vi "CD Init_Prepare Inline Data_Complete Frame Descriptors.vi"(8 "error in (no error)":errorcluster, 10 "RTs In":T1[](array[typedef]) {"Mode Codes"."Words Item Refs" format="%.0x"; "Mode Codes"."Words Block Data Refs"."Data Reference" format="%.0x"; "Mode Codes"."Timestamp Channel Data Reference" format="%.0x"; "subAddresses"."Words Item Refs" format="%.0x"; "subAddresses"."Words Block Data Refs"."Data Reference" format="%.0x"; "subAddresses"."Timestamp Channel Data Reference" format="%.0x"; "Status Channel Data Reference" format="%.0x"; "Command Channels Refs" format="%.0x"}, 11 "Frames Descriptors In":T9[](array[typedef]) {"RT"."Status Channel Ref" format="%.0x"; "RT"."Words Block Data Refs"."Data Reference" format="%.0x"; "RT"."Timestamp Channel Data Reference" format="%.0x"; "BC"."Status Channel Refs" format="%.0x"; "BC"."Words Block Data Refs"."Data Reference" format="%.0x"; "BC"."Timestamp Channel Data Reference" format="%.0x"}) -> (0 "error out":errorcluster, 3 "Frames Descriptors Out":T9[](array[typedef]) {"RT"."Status Channel Ref" format="%.0x"; "RT"."Words Block Data Refs"."Data Reference" format="%.0x"; "RT"."Timestamp Channel Data Reference" format="%.0x"; "BC"."Status Channel Refs" format="%.0x"; "BC"."Words Block Data Refs"."Data Reference" format="%.0x"; "BC"."Timestamp Channel Data Reference" format="%.0x"})   [LabVIEW 2017, in "Ballard MIL-1553 Engine.lvlib"]
doc: "We complete Frame Descriptors for frames not defined in BC (or there is no BC)."
uses:
  Ballard MIL-1553 Engine.lvlib
  Controls/RT Inline Frame Descriptor.ctl
  Controls/RT Inline Frame Descriptor_BC.ctl
  <vilib>/NI Veristand/Custom Device API/Data Reference.ctl
  <vilib>/NI Veristand/Custom Device API/Block Data Reference.ctl
  <vilib>/NI Veristand/Custom Device API/Custom Device Item Ref.ctl
  Controls/RT Inline Frame Descriptor_RT.ctl
  Shared/Controls and Global/RT CWD2.ctl
  Shared/Controls and Global/RT CWD1.ctl
  Shared/Controls and Global/RT messageType.ctl
  Shared/Controls and Global/RT Remote Terminal.ctl
  Shared/Controls and Global/RT Remote Terminal_rtMode.ctl
  Shared/Controls and Global/RT Remote Terminal_RT subAddress.ctl
  Shared/Controls and Global/RT Remote Terminal_RT direction.ctl
  Shared/Controls and Global/RT Remote Terminal_RT Mode Code.ctl
  <vilib>/NI VeriStand/Custom Device Tools/Custom Device Utility Library/Custom Device Utility Library.lvlib
  Shared/Ballard 1553 Shared.lvlib
  <vilib>/NI VeriStand/Custom Device API/Custom Device API.lvlib
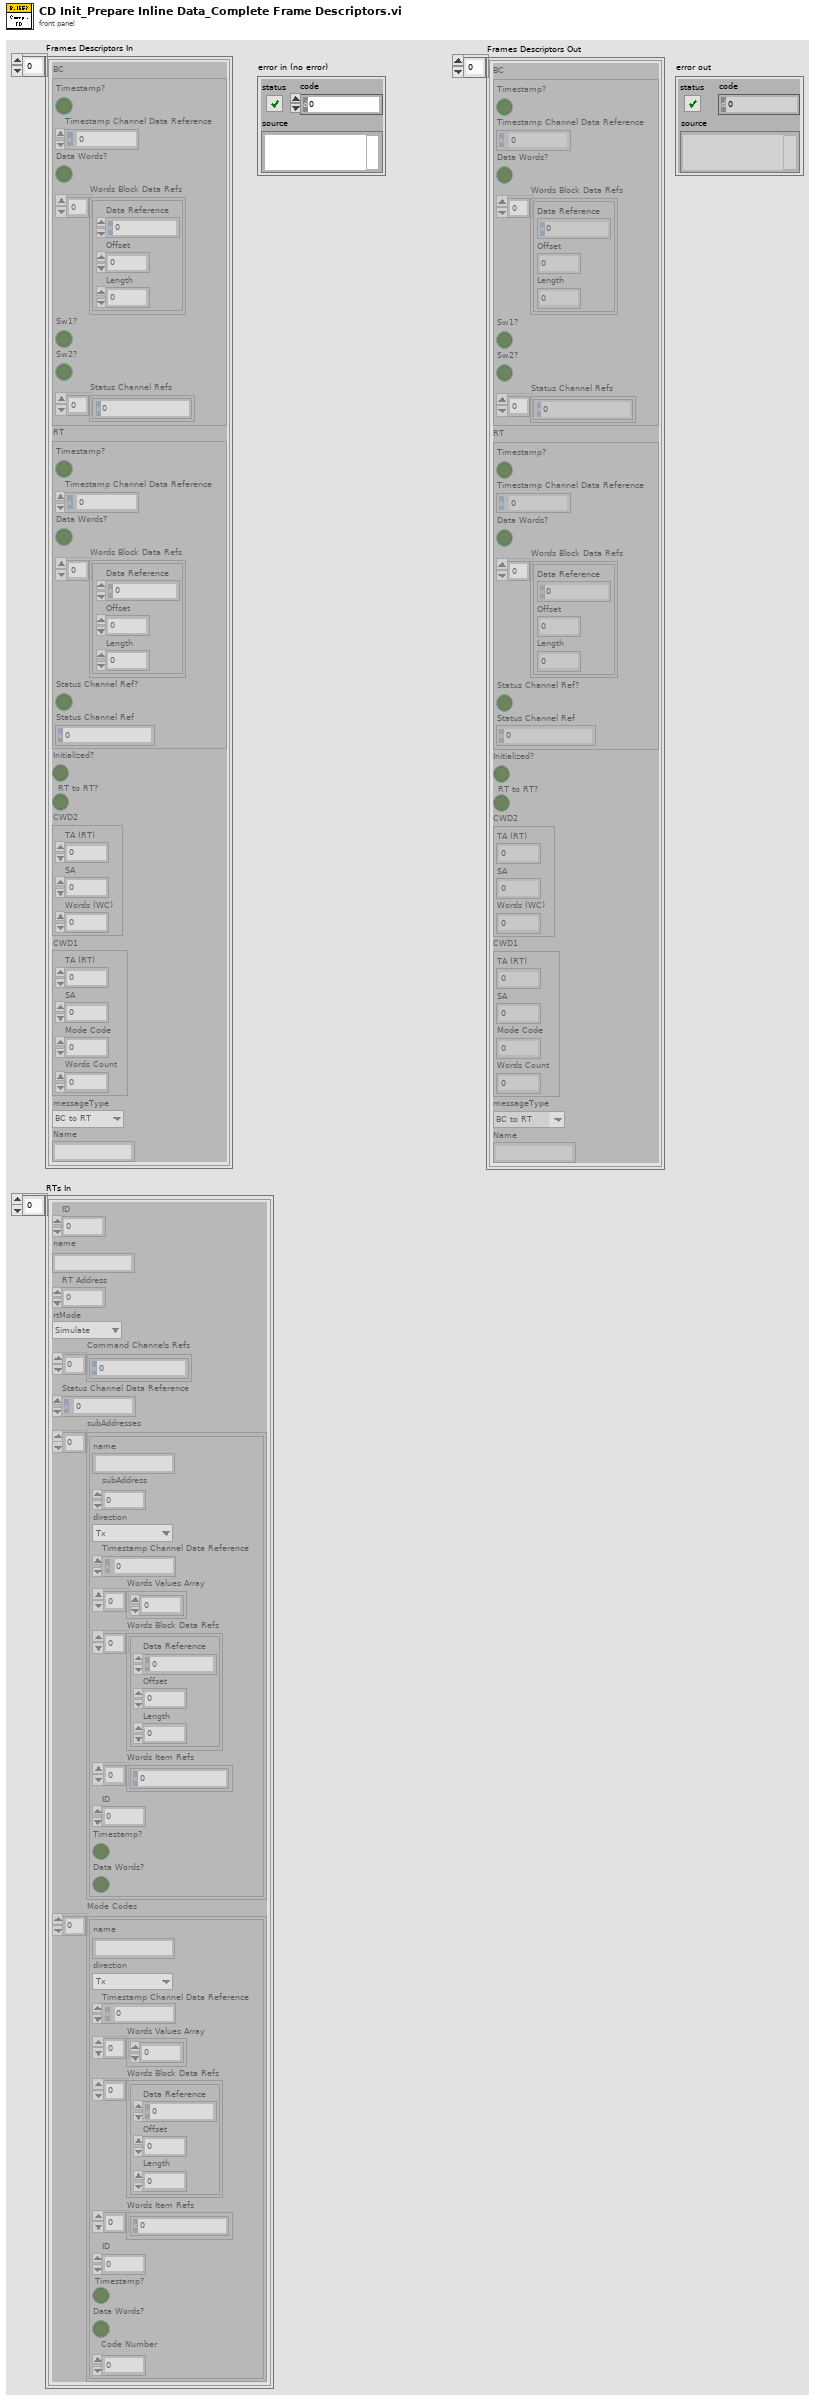
[diagram p1: front panel]
types:
  T1 = typedef "Ballard 1553 Shared.lvlib/RT Remote Terminal.ctl" = cluster{"ID":i32, "name":string, "RT Address":i32, "rtMode":T2, "Command Channels Refs":T3[], "Status Channel Data Reference":T4, "subAddresses":T5[], "Mode Codes":T8[]}
  T2 = typedef "Ballard 1553 Shared.lvlib/RT Remote Terminal_rtMode.ctl" = enum16{"Simulate", "Monitor", "Disable"}
  T3 = typedef "Custom Device API.lvlib/Custom Device Item Ref.ctl" = u64
  T4 = typedef "Custom Device API.lvlib/Data Reference.ctl" = i32
  T5 = typedef "Ballard 1553 Shared.lvlib/RT Remote Terminal_RT subAddress.ctl" = cluster{"name":string, "subAddress":i8, "direction":T6, "Timestamp Channel Data Reference":T4, "Words Values Array":u16[], "Words Block Data Refs":T7[], "Words Item Refs":T3[], "ID":i32, "Timestamp?":bool, "Data Words?":bool}
  T6 = typedef "Ballard 1553 Shared.lvlib/RT Remote Terminal_RT direction.ctl" = enum16{"Tx", "Rx"}
  T7 = typedef "Custom Device API.lvlib/Block Data Reference.ctl" = cluster{"Data Reference":T4, "Offset":u64, "Length":u64}
  T8 = typedef "Ballard 1553 Shared.lvlib/RT Remote Terminal_RT Mode Code.ctl" = cluster{"name":string, "direction":T6, "Timestamp Channel Data Reference":T4, "Words Values Array":u16[], "Words Block Data Refs":T7[], "Words Item Refs":T3[], "ID":i32, "Timestamp?":bool, "Data Words?":bool, "Code Number":i32}
  T9 = typedef "Ballard MIL-1553 Engine.lvlib/RT Inline Frame Descriptor.ctl" = cluster{"BC":T10, "RT":T11, "Initialized?":bool, "RT to RT?":bool, "CWD2":T12, "CWD1":T13, "messageType":T14, "Name":string}
  T10 = typedef "Ballard MIL-1553 Engine.lvlib/RT Inline Frame Descriptor_BC.ctl" = cluster{"Timestamp?":bool, "Timestamp Channel Data Reference":T4, "Data Words?":bool, "Words Block Data Refs":T7[], "Sw1?":bool, "Sw2?":bool, "Status Channel Refs":T3[]}
  T11 = typedef "Ballard MIL-1553 Engine.lvlib/RT Inline Frame Descriptor_RT.ctl" = cluster{"Timestamp?":bool, "Timestamp Channel Data Reference":T4, "Data Words?":bool, "Words Block Data Refs":T7[], "Status Channel Ref?":bool, "Status Channel Ref":T3}
  T12 = typedef "Ballard 1553 Shared.lvlib/RT CWD2.ctl" = cluster{"TA (RT)":i8, "SA":i8, "Words (WC)":i8}
  T13 = typedef "Ballard 1553 Shared.lvlib/RT CWD1.ctl" = cluster{"TA (RT)":i8, "SA":i8, "Mode Code":i8, "Words Count":i8}
  T14 = typedef "Ballard 1553 Shared.lvlib/RT messageType.ctl" = enum16{"BC to RT", "RT to BC", "RT to RT", "MC (Rx)", "MC (Tx)"}
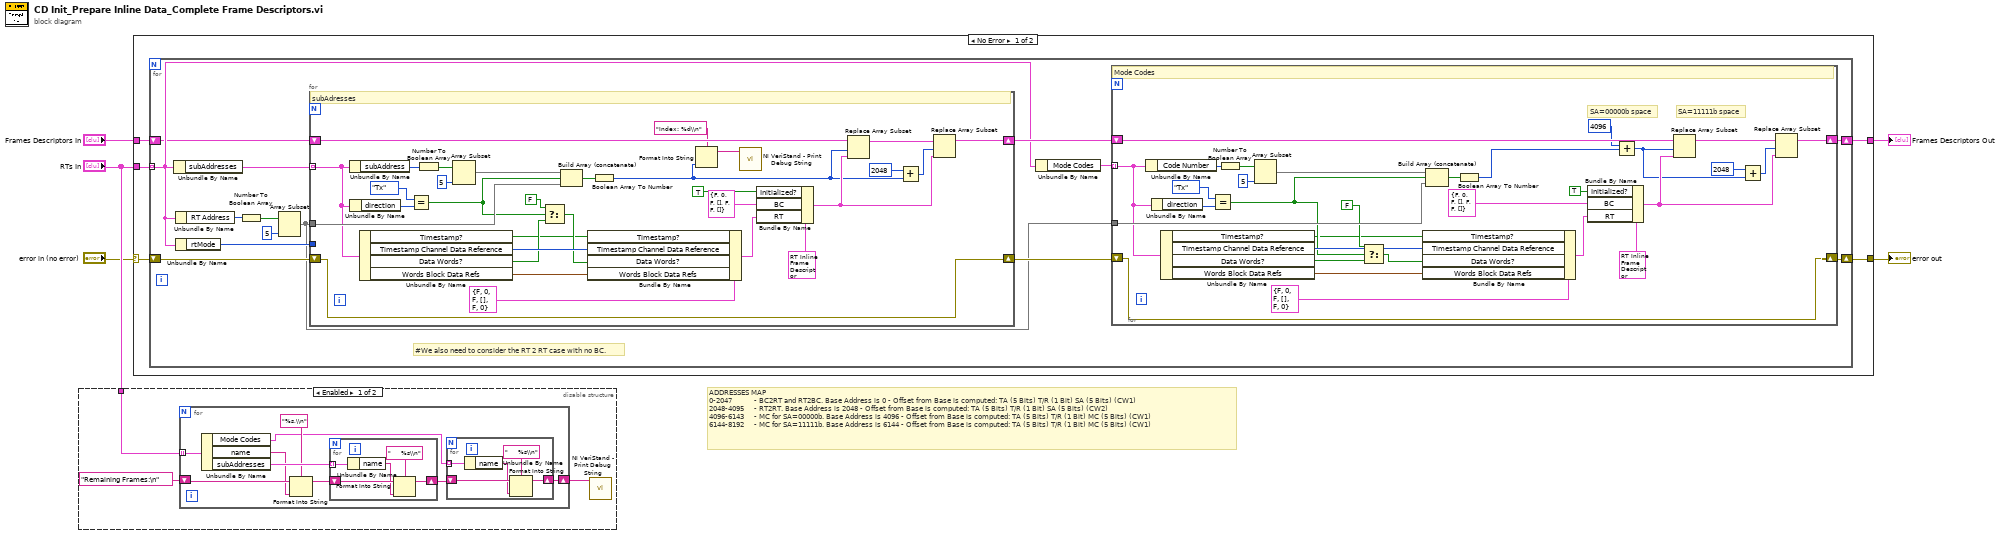
[diagram p0: block diagram]
diagram:
  # "ADDRESSES MAP \n0-2047           - BC2RT and RT2BC. Base Address is 0 - Offset from Base is computed: TA (5 Bits) T/R (1 Bit) SA (5 Bits) (CW1)\n2048-4095     - RT2RT. Base Address is 2048 - Offset from Base is computed: TA (5 Bits) T/R (1 Bit) SA (5 Bits) (CW2)\n4096-6143     - MC for SA=00000b. Base Address is 4096 - Offset from Base is computed: TA (5 Bits) T/R (1 Bit) MC (5 Bits) (CW1)\n6144-8192     - MC for SA=11111b. Base Address is 6144 - Offset from Base is computed: TA (5 Bits) T/R (1 Bit) MC (5 Bits) (CW1)"
  n1 = disable-structure shown="Enabled" {
    disable-tunnel: "RTs In" -> [w8 _]
    frame Enabled {
      n2 = for {
        tunnel: w8 -> [w17] mode=indexing
        shift-right: [w11] -> w6
        shift-left: "Remaining Frames:\n" -> [w15]
        n3 = Unbundle By Name(w17) -> ("Mode Codes"=w9:T8[], "name"=w14:string, "subAddresses"=w16:T5[])
        n4 = Format Into String(format string="%s,\\n", initial string=w15, w14) -> (resulting string=w12:string)  [unwired: 1 in, 1 out]
        n5 = for {
          tunnel: w16 -> [w27] mode=indexing
          shift-right: [w26] -> w10
          shift-left: w12 -> [w25]
          n6 = Unbundle By Name(w27) -> ("name"=w24:string)
          n7 = Format Into String(format string="     %s\\n", initial string=w25, w24) -> (resulting string=w26:string)  [unwired: 1 in, 1 out]
        }
        n8 = for {
          tunnel: w9 -> [w22] mode=indexing
          shift-right: [w21] -> w11
          shift-left: w10 -> [w20]
          n9 = Unbundle By Name(w22) -> ("name"=w19:string)
          n10 = Format Into String(format string="     %s\\n", initial string=w20, w19) -> (resulting string=w21:string)  [unwired: 1 in, 1 out]
        }
      }
      n11 = call <vilib>:"NI VeriStand - Print Debug String.vi"("Message"=w6) -> ()  [unwired: 10 in, 1 out]
    }
    frame Disabled {
    }
  }
  n12 = case shown="No Error" "error in (no error)" {
    selector: "error in (no error)" -> [w28 w110]
    tunnel: [w32 w109] -> w5
    tunnel: "Frames Descriptors In" -> [w31 w109]
    tunnel: [w30 w110] -> w3
    tunnel: "RTs In" -> [w29 _]
    frame No Error {
      n13 = for {
        tunnel: w29 -> [w36] mode=indexing
        shift-right: [w39] -> w32
        shift-left: w31 -> [w33]
        shift-right: [w37] -> w30
        shift-left: w28 -> [w41]
        # "#We also need to consider the RT 2 RT case with no BC."
        n14 = Unbundle By Name(w36) -> ("subAddresses"=w43:T5[])
        n15 = Unbundle By Name(w36) -> ("RT Address"=w44:i32)
        n16 = Unbundle By Name(w36) -> ("rtMode"=w42:T2)
        n17 = Number To Boolean Array(number=w44) -> (Boolean array=w45:bool[])
        n18 = Array Subset(array=w45, length=5) -> (w34:bool[])  [unwired: 1 in]
        n19 = for {
          tunnel: w34 -> [w101]
          shift-right: [w92] -> w40
          shift-left: w33 -> [w89]
          tunnel: w43 -> [w96] mode=indexing
          tunnel: w42 -> [_]
          shift-right: [w90] -> w38
          shift-left: w41 -> [w90]
          # "subAdresses"
          n20 = Unbundle By Name(w96) -> ("subAddress"=w106:i8)
          n21 = Unbundle By Name(w96) -> ("direction"=w103:T6)
          n22 = Unbundle By Name(w96) -> ("Timestamp?"=w82:bool, "Timestamp Channel Data Reference"=w94:T4, "Data Words?"=w84:bool, "Words Block Data Refs"=w93:T7[])
          n23 = Equal?(x=RT_Remote_Terminal_RT_direction."Tx", y=w103) -> (x = y?=w86:bool)
          n24 = Number To Boolean Array(number=w106) -> (Boolean array=w107:bool[])
          n25 = Array Subset(array=w107, length=5) -> (w104:bool[])  [unwired: 1 in]
          n26 = Select(t=FALSE, s=w86, f=w84) -> (s? t:f=w83:bool)
          n27 = Build Array (concatenate)(w104, w86, w101) -> (w105:bool[])
          n28 = Bundle By Name(cluster=T11 {"Timestamp?"=FALSE, "Timestamp Channel Data Reference"=0, "Data Words?"=FALSE, "Words Block Data Refs"=[], "Status Channel Ref?"=FALSE, "Status Channel Ref"=0} ("RT"), "Timestamp?"=w82, "Timestamp Channel Data Reference"=w94, "Data Words?"=w83, "Words Block Data Refs"=w93) -> (w95:T11)
          n29 = Boolean Array To Number(Boolean array=w105) -> (number=w78:u16)
          n30 = Format Into String(format string="Index: %d\\n", w78) -> (resulting string=w80:string)  [unwired: 2 in, 1 out]
          n31 = call <vilib>:"NI VeriStand - Print Debug String.vi"("Message"=w80) -> ()  [unwired: 10 in, 1 out]
          n32 = Bundle By Name(cluster=T9 {"BC"={"Timestamp?"=FALSE, "Timestamp Channel Data Reference"=0, "Data Words?"=FALSE, "Words Block Data Refs"=[], "Sw1?"=FALSE, "Sw2?"=FALSE, "Status Channel Refs"=[]}, "RT"={"Timestamp?"=FALSE, "Timestamp Channel Data Reference"=0, "Data Words?"=FALSE, "Words Block Data Refs"=[], "Status Channel Ref?"=FALSE, "Status Channel Ref"=0}, "Initialized?"=FALSE, "RT to RT?"=FALSE, "CWD2"={"TA (RT)"=0, "SA"=0, "Words (WC)"=0}, "CWD1"={"TA (RT)"=0, "SA"=0, "Mode Code"=0, "Words Count"=0}, "messageType"=enum."BC to RT", "Name"=""} ("Frame Descriptor"), "Initialized?"=TRUE, "BC"=T10 {"Timestamp?"=FALSE, "Timestamp Channel Data Reference"=0, "Data Words?"=FALSE, "Words Block Data Refs"=[], "Sw1?"=FALSE, "Sw2?"=FALSE, "Status Channel Refs"=[]}, "RT"=w95) -> (w91:T9)
          n33 = Replace Array Subset(array=w89, new element=w91, index=w78) -> (w87:T9[])
          n34 = Add(x=u16 2048, y=w78) -> (x+y=w79:u16)
          n35 = Replace Array Subset(array=w87, new element=w91, index=w79) -> (w92:T9[])
        }
        n36 = Unbundle By Name(w36) -> ("Mode Codes"=w35:T8[])
        n37 = for {
          tunnel: w34 -> [w70]
          shift-right: [w60] -> w39
          shift-left: w40 -> [w69]
          tunnel: w35 -> [w64] mode=indexing
          shift-right: [w57] -> w37
          shift-left: w38 -> [w57]
          # "SA=11111b space"
          # "SA=00000b space"
          # "Mode Codes"
          n38 = Unbundle By Name(w64) -> ("Code Number"=w75:i32)
          n39 = Unbundle By Name(w64) -> ("direction"=w72:T6)
          n40 = Unbundle By Name(w64) -> ("Timestamp?"=w47:bool, "Timestamp Channel Data Reference"=w62:T4, "Data Words?"=w48:bool, "Words Block Data Refs"=w61:T7[])
          n41 = Equal?(x=RT_Remote_Terminal_RT_direction."Tx", y=w72) -> (x = y?=w51:bool)
          n42 = Number To Boolean Array(number=w75) -> (Boolean array=w76:bool[])
          n43 = Array Subset(array=w76, length=5) -> (w73:bool[])  [unwired: 1 in]
          n44 = Select(t=FALSE, s=w51, f=w48) -> (s? t:f=w49:bool)
          n45 = Bundle By Name(cluster=T11 {"Timestamp?"=FALSE, "Timestamp Channel Data Reference"=0, "Data Words?"=FALSE, "Words Block Data Refs"=[], "Status Channel Ref?"=FALSE, "Status Channel Ref"=0} ("RT"), "Timestamp?"=w47, "Timestamp Channel Data Reference"=w62, "Data Words?"=w49, "Words Block Data Refs"=w61) -> (w63:T11)
          n46 = Build Array (concatenate)(w73, w51, w70) -> (w74:bool[])
          n47 = Boolean Array To Number(Boolean array=w74) -> (number=w58:u16)
          n48 = Bundle By Name(cluster=T9 {"BC"={"Timestamp?"=FALSE, "Timestamp Channel Data Reference"=0, "Data Words?"=FALSE, "Words Block Data Refs"=[], "Sw1?"=FALSE, "Sw2?"=FALSE, "Status Channel Refs"=[]}, "RT"={"Timestamp?"=FALSE, "Timestamp Channel Data Reference"=0, "Data Words?"=FALSE, "Words Block Data Refs"=[], "Status Channel Ref?"=FALSE, "Status Channel Ref"=0}, "Initialized?"=FALSE, "RT to RT?"=FALSE, "CWD2"={"TA (RT)"=0, "SA"=0, "Words (WC)"=0}, "CWD1"={"TA (RT)"=0, "SA"=0, "Mode Code"=0, "Words Count"=0}, "messageType"=enum."BC to RT", "Name"=""} ("Frame Descriptor"), "Initialized?"=TRUE, "BC"=T10 {"Timestamp?"=FALSE, "Timestamp Channel Data Reference"=0, "Data Words?"=FALSE, "Words Block Data Refs"=[], "Sw1?"=FALSE, "Sw2?"=FALSE, "Status Channel Refs"=[]}, "RT"=w63) -> (w59:T9)
          n49 = Add(x=u16 4096, y=w58) -> (x+y=w55:u16)
          n50 = Replace Array Subset(array=w69, new element=w59, index=w55) -> (w56:T9[])
          n51 = Add(x=u16 2048, y=w55) -> (x+y=w53:u16)
          n52 = Replace Array Subset(array=w56, new element=w59, index=w53) -> (w60:T9[])
        }
      }
    }
    frame Error {
    }
  }
  "Frames Descriptors Out" <- w5
  "error out" <- w3
